vi "CreatePrivateEvents.vi"(8 "error in (no error)":errorcluster, 11 "MAUI":refnum<class "MAUI.lvclass">) -> (0 "error out":errorcluster, 3 "MAUI out":refnum<class "MAUI.lvclass">)   [LabVIEW 2016, in "MAUI.lvclass"]
doc: "---------------------------------------------------------------\nJKI State Machine Objects™\nhttp://jki.net/state-machine-objects/\nCopyright (C) 2005-2015, JKI <info@jki.net>\nALL RIGHTS RESERVEDJKI State Machine Objects (SMO) 1.0.0.4\nJKI - JKI\nCopyright (c) 2015, JKI"
uses:
  MAUI.lvclass
  Typedefs/PrivateEvents--MAUI.SetLeftData.ctl
  Typedefs/PrivateEvents--MAUI.SetRightData.ctl
  Typedefs/PrivateEvents--MAUI.GetRightData.ctl
  Typedefs/PanelData.ctl
  Typedefs/PrivateEvents--MAUI.GetLeftData.ctl
  Typedefs/PanelDataNotifier.ctl
  Typedefs/PrivateEvents--MAUI.SetEmbedded.ctl
  <vilib>/Levylab/Embedded SMO UI/EmbeddedSMO.lvclass
  Typedefs/PrivateEvents--MAUI.GetEmbedded.ctl
  Typedefs/PrivateEvents--MAUI.Update Left Subpanel.ctl
  Typedefs/PrivateEvents--MAUI.UpdateRightSubpanel.ctl
  MAUI.lvclass/MAUI.ctl
  <vilib>/JKI/JKI SMO/SMO.UI/SMO.UI.lvclass
panel:
  # "For instructions on how to use the JKI State Machine Objects, examples and video tutorials, visit:\nhttp://jki.net/state-machine-objects/\n\nJKI State Machine Objects™\nhttp://jki.net/state-machine-objects/\nCopyright (C) 2005-2015, JKI <info@jki.net>\nALL RIGHTS RESERVED"
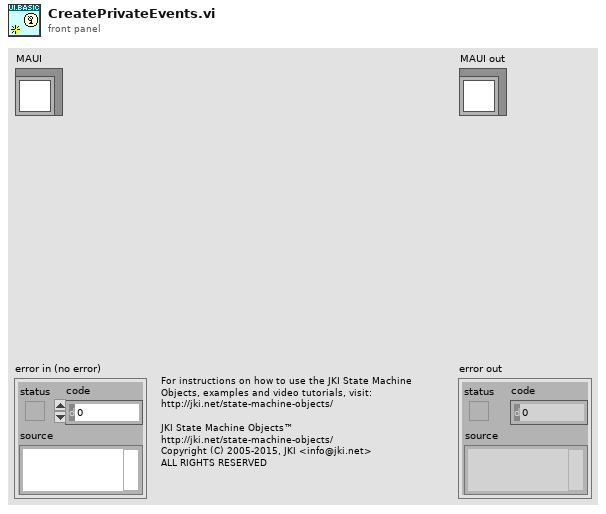
[diagram p1: front panel]
types:
  T1 = typedef "MAUI.lvclass/PrivateEvents--MAUI.UpdateRightSubpanel.ctl" = i32
  T2 = typedef "MAUI.lvclass/PrivateEvents--MAUI.Update Left Subpanel.ctl" = i32
  T3 = typedef "MAUI.lvclass/PrivateEvents--MAUI.GetEmbedded.ctl" = cluster{"notifier out":refnum<notifier>}
  T4 = typedef "MAUI.lvclass/PrivateEvents--MAUI.SetEmbedded.ctl" = cluster{"Subpanels":refnum<class "EmbeddedSMO.lvclass">[]}
  T5 = typedef "MAUI.lvclass/PrivateEvents--MAUI.GetLeftData.ctl" = cluster{"notifier":T6}
  T6 = typedef "MAUI.lvclass/PanelDataNotifier.ctl" = refnum<notifier>
  T7 = typedef "MAUI.lvclass/PrivateEvents--MAUI.GetRightData.ctl" = cluster{"notifier":refnum<notifier>}
  T8 = typedef "MAUI.lvclass/PrivateEvents--MAUI.SetRightData.ctl" = cluster{"Right":cluster{"Subpanel":refnum<vi>, "Ring":refnum<vi>, "Active":i32}}
  T9 = typedef "MAUI.lvclass/PrivateEvents--MAUI.SetLeftData.ctl" = cluster{"Left":cluster{"Subpanel":refnum<vi>, "Ring":refnum<vi>, "Active":i32}}
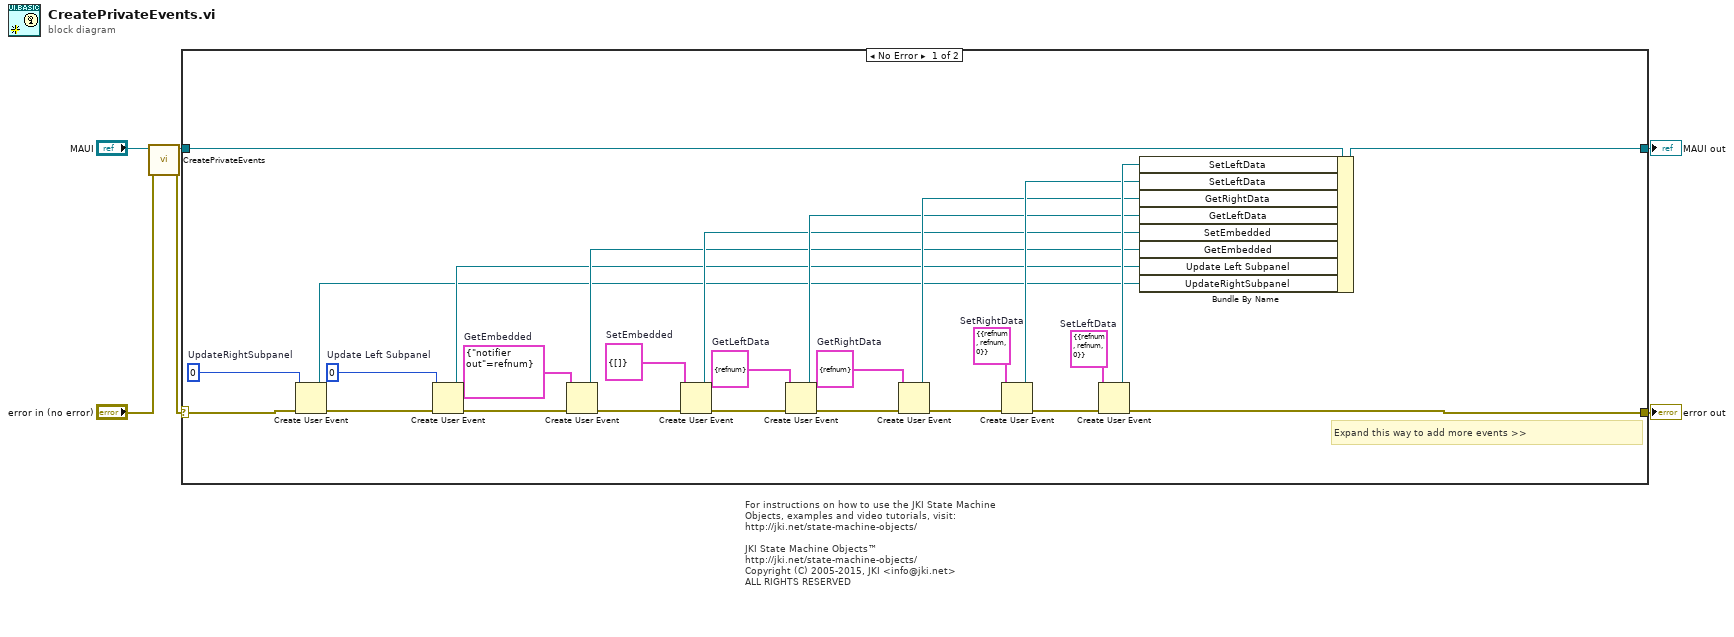
[diagram p0: block diagram]
diagram:
  # "For instructions on how to use the JKI State Machine Objects, examples and video tutorials, visit:\nhttp://jki.net/state-machine-objects/\n\nJKI State Machine Objects™\nhttp://jki.net/state-machine-objects/\nCopyright (C) 2005-2015, JKI <info@jki.net>\nALL RIGHTS RESERVED"
  n1 = call-parent "CreatePrivateEvents.vi"("error in (no error)"="error in (no error)", "SMO.UI"="MAUI") -> ("error out"=w1:errorcluster, "SMO.UI out"=w3:refnum<class "MAUI.lvclass">)  [unwired: 8 in]
  n2 = case shown="No Error" w1 {
    selector: w1 -> [w32 w35]
    tunnel: [w30 w35] -> w5
    tunnel: [w31 w34] -> w6
    tunnel: w3 -> [w33 w34]
    frame No Error {
      w8 = T1 0  # UpdateRightSubpanel
      w11 = T2 0  # Update Left Subpanel
      w14 = T3 {"notifier out"=refnum}  # GetEmbedded
      w17 = T4 {"Subpanels"=[]}  # SetEmbedded
      w20 = T5 {"notifier"=refnum}  # GetLeftData
      w23 = T7 {"notifier"=refnum}  # GetRightData
      w26 = T8 {"Right"={"Subpanel"=refnum, "Ring"=refnum, "Active"=0}}  # SetRightData
      w29 = T9 {"Left"={"Subpanel"=refnum, "Ring"=refnum, "Active"=0}}  # SetLeftData
      # "Expand this way to add more events >>"
      n3 = Create User Event(user event datatype=w8, error in=w32) -> (user event=w7:refnum<user-event>, error out=w9:errorcluster)
      n4 = Create User Event(user event datatype=w11, error in=w9) -> (user event=w10:refnum<user-event>, error out=w12:errorcluster)
      n5 = Create User Event(user event datatype=w14, error in=w12) -> (user event=w13:refnum<user-event>, error out=w15:errorcluster)
      n6 = Create User Event(user event datatype=w17, error in=w15) -> (user event=w16:refnum<user-event>, error out=w18:errorcluster)
      n7 = Create User Event(user event datatype=w20, error in=w18) -> (user event=w19:refnum<user-event>, error out=w21:errorcluster)
      n8 = Create User Event(user event datatype=w23, error in=w21) -> (user event=w22:refnum<user-event>, error out=w24:errorcluster)
      n9 = Create User Event(user event datatype=w26, error in=w24) -> (user event=w25:refnum<user-event>, error out=w27:errorcluster)
      n10 = Create User Event(user event datatype=w29, error in=w27) -> (user event=w28:refnum<user-event>, error out=w30:errorcluster)
      n11 = Bundle By Name(cluster=w33, "SetLeftData"=w28, "SetLeftData"=w25, "GetRightData"=w22, "GetLeftData"=w19, "SetEmbedded"=w16, "GetEmbedded"=w13, "Update Left Subpanel"=w10, "UpdateRightSubpanel"=w7) -> (w31:refnum<class "MAUI.lvclass">)
    }
    frame Error {
    }
  }
  "error out" <- w5
  "MAUI out" <- w6
